vi "SingleConnection.vi"() -> ()   [LabVIEW 2016]
doc: "This VI acts as a server for an incoming websockets connection. Receives/sends string data to the connected client.\nWebSockets 1.6.0.22\nSam Sharp - MediaMongrels Ltd\nCopyright (c) 2016, MediaMongrels Ltd"
uses:
  WebSockets/WebSockets.lvlib
panel:
  in  "Resource Names":string[](array[string])
  out "Host":string
  out "Resource Name":string
  out "Request URI":string
  out "HTTP Headers":variant
  in  "Stop":bool
  out "Received Data":string
  in  "Send":bool
  in  "Data":string
  # "WebSockets Example Server"
  # "This VI is a simple example of sending/receiving data using WebSockets.\nIt waits for a single incoming WebSockets connection on Port 6123 and\nthen displays incoming string data. Strings can also be sent back to the client.\n\nInstructions for use:\n1) Run this VI\n2) Open the index.html file located in the examples folder\n3) The index.html will display the status of the connection and once established, data can be sent/received from either this VI or the index.html file."
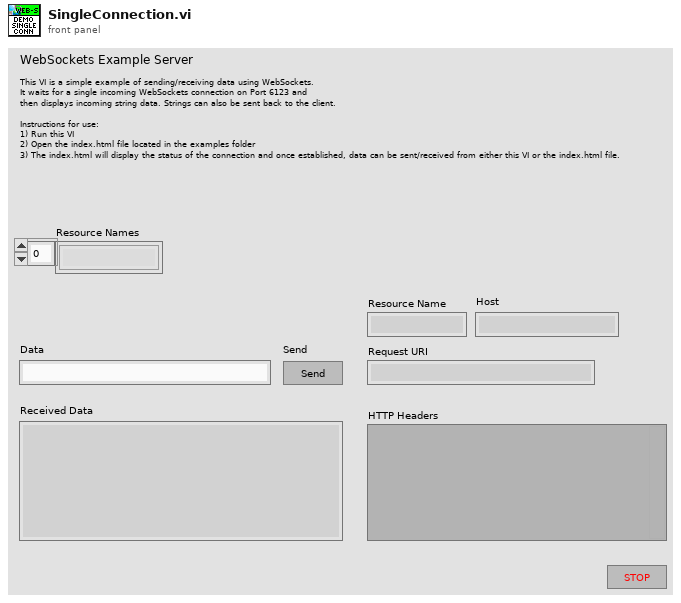
[diagram p1: front panel]
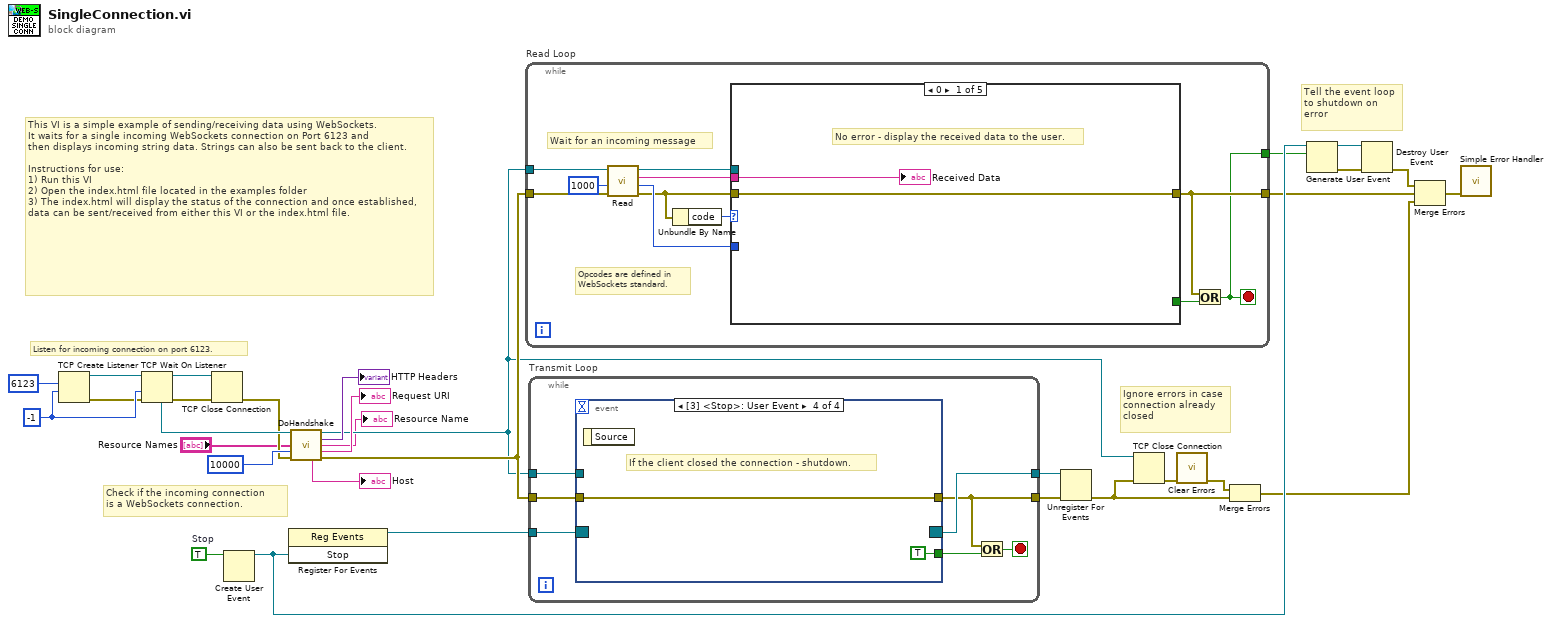
[diagram p0: block diagram]
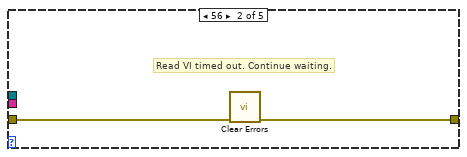
[diagram p2: hidden frame]
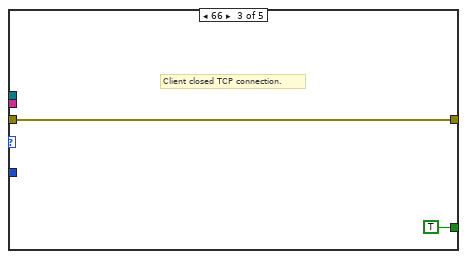
[diagram p3: hidden frame]
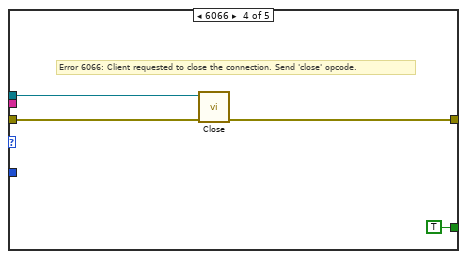
[diagram p4: hidden frame]
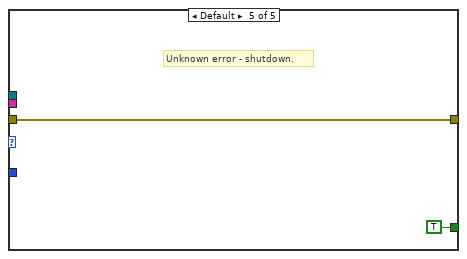
[diagram p5: hidden frame]
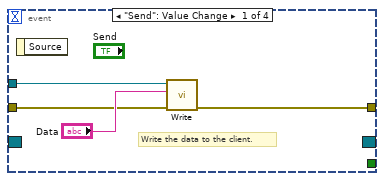
[diagram p6: hidden frame]
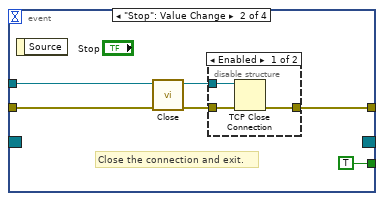
[diagram p7: hidden frame]
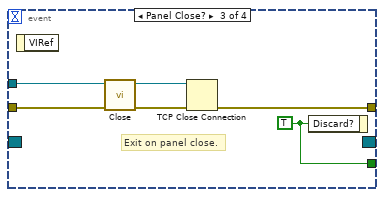
[diagram p9: hidden frame]
diagram:
  w23 = TRUE  # Stop
  w30 = -1 ("timeout ms (25000)")
  # "Ignore errors in case\nconnection already\nclosed"
  # "Tell the event loop to shutdown on error"
  # "This VI is a simple example of sending/receiving data using WebSockets.\nIt waits for a single incoming WebSockets connection on Port 6123 and\nthen displays incoming string data. Strings can also be sent back to the client.\n\nInstructions for use:\n1) Run this VI\n2) Open the index.html file located in the examples folder\n3) The index.html will display the status of the connection and once established, data can be sent/received from either this VI or the index.html file."
  # "Check if the incoming connection\nis a WebSockets connection."
  # "Listen for incoming connection on port 6123."
  n1 = TCP Create Listener(9:w30, 10:u16 6123 ("port")) -> (0:w28:errorcluster, 3:w29:refnum<k5>)  [unwired: 3 in, 1 out]
  n2 = TCP Wait On Listener(8:w28, 9:w30, 11:w29) -> (0:w25:errorcluster, 3:w26:refnum<k5>, 4:w27:refnum<k5>)  [unwired: 1 in, 2 out]
  n3 = TCP Close Connection(connection ID=w26, error in (no error)=w25) -> (error out=w3:errorcluster)  [unwired: 1 in, 1 out]
  n4 = Create User Event(user event datatype=w23) -> (user event=w21:refnum<user-event>)  [unwired: 1 in, 1 out]
  n5 = register-events(w21) -> (reference out=w24:refnum<event-registration>)  [unwired: 2 in, 1 out]
  n6 = call "DoHandshake.vi"("WebSocket Connection in"=w27, "Resource Names"="Resource Names", "timeout ms (5000)"=10000 ("timeout ms (25000)"), "error in (no error)"=w3) -> ("WebSocket Connection out"=w9:refnum<k5>, "Headers Out"=→"HTTP Headers":variant, "Resource Name"=→"Resource Name":string, "Request URI"=→"Request URI":string, "Host"=→"Host":string, "error out"=w11:errorcluster)  [unwired: 6 in]
  n7 = while "Read Loop" {
    tunnel: w9 -> [w42]
    tunnel: [w32] -> w20
    tunnel: [w34] -> w10
    tunnel: w11 -> [w35]
    stop <- w32 stop-if-true
    # "Wait for an incoming message"
    # "Opcodes are defined in\nWebSockets standard."
    n8 = call "Read.vi"("error in (no error)"=w35, "timeout ms (5000)"=1000 ("timeout ms (25000)"), "WebSocket Connection in"=w42) -> ("error out"=w36:errorcluster, "Opcode"=w37:u8, "Data"=w39:string, "WebSocket Connection out"=w38:refnum<k5>)  [unwired: 5 in]
    n9 = Unbundle By Name(w36) -> ("code"=w40:i32)
    n10 = case shown="0" w40 {
      tunnel: w39 -> [w44 _ _ _ _]
      tunnel: [_ _ TRUE TRUE TRUE] -> w33
      tunnel: w38 -> [_ _ _ w52 _]
      tunnel: w37 -> [_ _ _ _ _]
      tunnel: w36 -> [w43 w46 w47 w50 w53]
      tunnel: [w43 w45 w47 w49 w53] -> w34
      frame 0 {
        # "No error - display the received data to the user."
        "Received Data" <- w44
      }
      frame 56 {
        # "Read VI timed out. Continue waiting."
        n11 = call <vilib>:"Clear Errors.vi"("error in (no error)"=w46) -> ("error out"=w45:errorcluster)  [unwired: 5 in, 1 out]
      }
      frame 66 {
        # "Client closed TCP connection."
      }
      frame 6066 {
        # "Error 6066: Client requested to close the connection. Send 'close' opcode."
        n12 = call "Close.vi"("error in (no error)"=w50, "WebSocket Connection in"=w52) -> ("error out"=w49:errorcluster)  [unwired: 8 in, 1 out]
      }
      frame Default {
        # "Unknown error - shutdown."
      }
    }
    n13 = Or(x=w34, y=w33) -> (x .or. y?=w32:bool)
  }
  n14 = while "Transmit Loop" {
    tunnel: w9 -> [w61]
    tunnel: w24 -> [w60]
    tunnel: [w59] -> w22
    tunnel: [w55] -> w12
    tunnel: w11 -> [w58]
    stop <- w56 stop-if-true
    n15 = event shown="[3] <Stop>: User Event" {
      selector: w60 -> [_ _ _ _]
      dyn-events: [_ _ _ _] -> w59
      timeout: _ -> [_ _ _ _]
      tunnel: w61 -> [w65 w70 w80 _]
      tunnel: [_ TRUE w78 TRUE] -> w57
      tunnel: [w62 w68 w76 w81] -> w55
      tunnel: w58 -> [w63 w66 w75 w81]
      event "Send": Value Change {
        # "Write the data to the client."
        n16 = event-data() -> ()  [unwired: 1 in, 1 out]
        n17 = call "Write.vi"("error in (no error)"=w63, "Data"="Data", "WebSocket Connection in"=w65) -> ("error out"=w62:errorcluster)  [unwired: 7 in, 1 out]
      }
      event "Stop": Value Change {
        # "Close the connection and exit."
        n18 = event-data() -> ()  [unwired: 1 in, 1 out]
        n19 = call "Close.vi"("error in (no error)"=w66, "WebSocket Connection in"=w70) -> ("error out"=w67:errorcluster, "WebSocket Connection in"=w69:refnum<k5>)  [unwired: 8 in]
        n20 = disable-structure shown="Enabled" {
          disable-tunnel: w69 -> [w74 _]
          disable-tunnel: [w73 _] -> w68
          disable-tunnel: w67 -> [w72 _]
          frame Enabled {
            n21 = TCP Close Connection(connection ID=w74, error in (no error)=w72) -> (error out=w73:errorcluster)  [unwired: 1 in, 1 out]
          }
          frame Disabled {
          }
        }
      }
      event Panel Close? {
        w78 = TRUE ("Discard?")
        # "Exit on panel close."
        n22 = event-data() -> ()  [unwired: 1 in, 1 out]
        n23 = call "Close.vi"("error in (no error)"=w75, "WebSocket Connection in"=w80) -> ("error out"=w77:errorcluster, "WebSocket Connection in"=w79:refnum<k5>)  [unwired: 8 in]
        n24 = TCP Close Connection(connection ID=w79, error in (no error)=w77) -> (error out=w76:errorcluster)  [unwired: 1 in, 1 out]
        n25 = event-data("Discard?"=w78) -> ()  [unwired: 1 in, 1 out]
      }
      event User Event {
        # "If the client closed the connection - shutdown."
        n26 = event-data() -> ()  [unwired: 1 in, 1 out]
      }
    }
    n27 = Or(x=w55, y=w57) -> (x .or. y?=w56:bool)
  }
  n28 = Unregister For Events(event registration refnum=w22, error in=w12) -> (error out=w7:errorcluster)
  n29 = TCP Close Connection(connection ID=w9, error in (no error)=w7) -> (error out=w8:errorcluster)  [unwired: 1 in, 1 out]
  n30 = call <vilib>:"Clear Errors.vi"("error in (no error)"=w8) -> ("error out"=w5:errorcluster)  [unwired: 5 in, 1 out]
  n31 = Merge Errors(w5, w7) -> (w6:errorcluster)
  n32 = Generate User Event(user event=w21, event data cluster=w20) -> (user event out=w19:refnum<user-event>, error out=w18:errorcluster)  [unwired: 2 in]
  n33 = Destroy User Event(user event=w19, error in=w18) -> (error out=w17:errorcluster)
  n34 = Merge Errors(w17, w10, w6) -> (w13:errorcluster)
  n35 = call <vilib>:"Simple Error Handler.vi"("error in (no error)"=w13) -> ()  [unwired: 4 in, 5 out]
